vi "NewProductDialog.vi"(8 "error in (no error)":errorcluster) -> (0 "error out":errorcluster, 1 "Cancelled?":bool, 3 "NewProduct":T1)   [LabVIEW 2022 SP3]
uses:
  #typedef_product.ctl
panel:
  in  "Cancel Button":bool
  in  "OK Button":bool
  in  "Product":T1
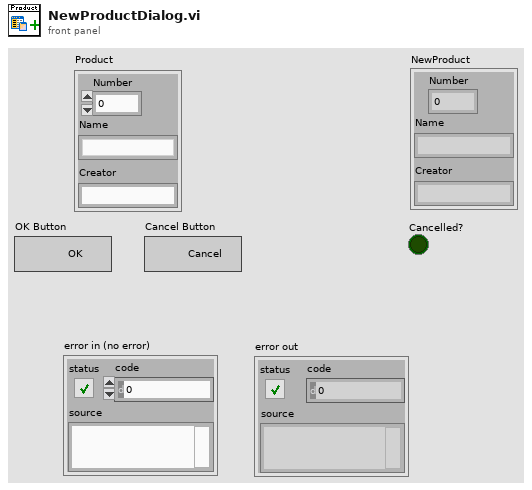
[diagram p1: front panel]
types:
  T1 = typedef "#typedef_product.ctl" = cluster{"Number ":dbl, "Name":string, "Creator":string}
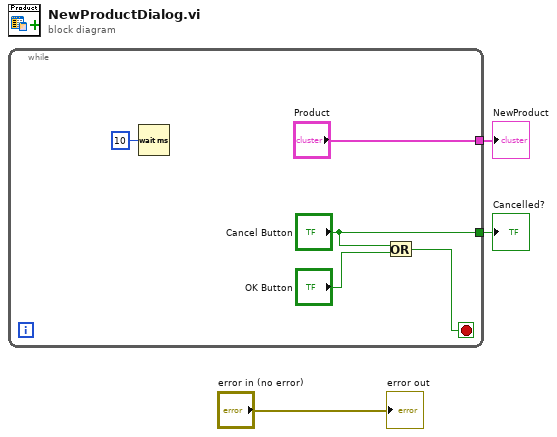
[diagram p0: block diagram]
diagram:
  n1 = while {
    tunnel: ["Product"] -> w3
    tunnel: ["Cancel Button"] -> w2
    stop <- w7 stop-if-true
    n2 = Wait (ms)(milliseconds to wait=u32 10) -> ()  [unwired: 1 out]
    n3 = Or(x="Cancel Button", y="OK Button") -> (x .or. y?=w7:bool)
  }
  "NewProduct" <- w3
  "Cancelled?" <- w2
  "error out" <- "error in (no error)"
